vi "FalconSwerveVelocityConversion.vi"(1 "Velocity (Raw Sensor Units per 100 ms)":i32) -> (0 "Velocity (ft/s)":dbl)   [LabVIEW 2020]
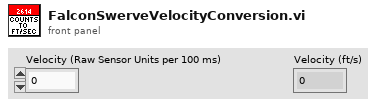
[diagram p1: front panel]
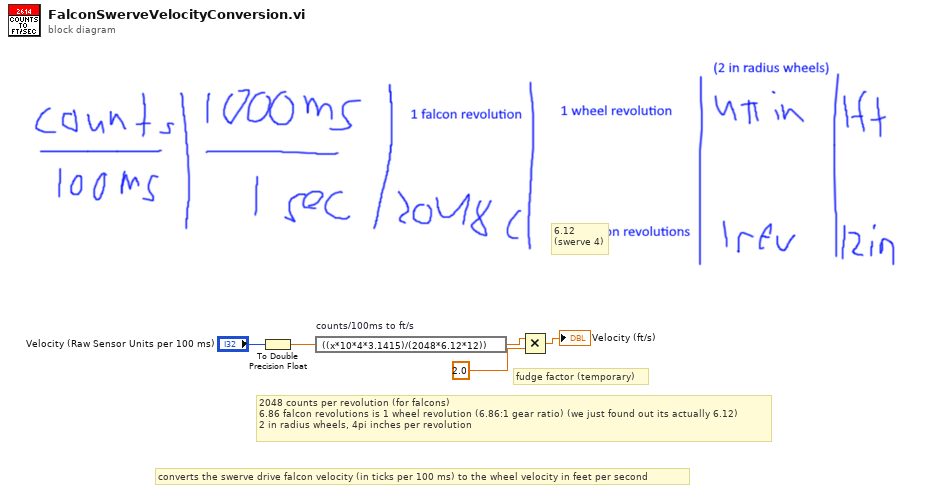
[diagram p0: block diagram]
diagram:
  # "fudge factor (temporary)"
  # "6.12\n(swerve 4)"
  # "converts the swerve drive falcon velocity (in ticks per 100 ms) to the wheel velocity in feet per second"
  # "2048 counts per revolution (for falcons)\n6.86 falcon revolutions is 1 wheel revolution (6.86:1 gear ratio) (we just found out its actually 6.12)\n2 in radius wheels, 4pi inches per revolution"
  n1 = To Double Precision Float(number="Velocity (Raw Sensor Units per 100 ms)") -> (double precision float=w4:dbl)
  n2 = expression code="((x*10*4*3.1415)/(2048*6.12*12))" "counts/100ms to ft/s"(w4) -> (w3:dbl)
  n3 = Multiply(x=w3, y=2.0) -> (x*y=→"Velocity (ft/s)":dbl)
